vi "Day 2 (Part Two).vi"() -> ()   [LabVIEW 2021]
panel:
  out "Score":i32
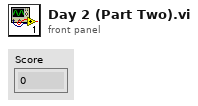
[diagram p1: front panel]
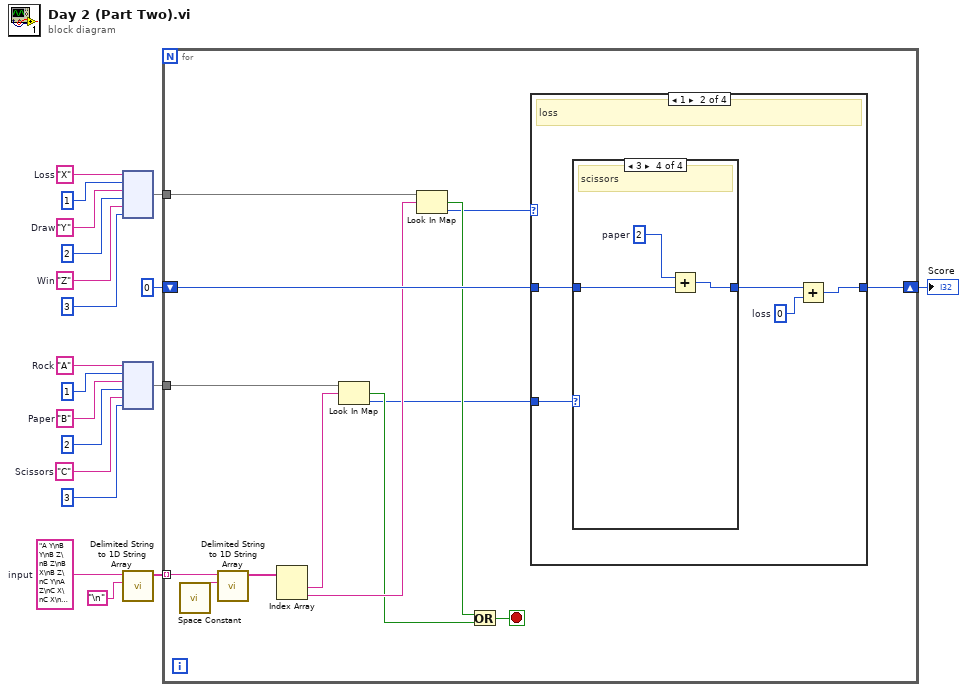
[diagram p0: block diagram]
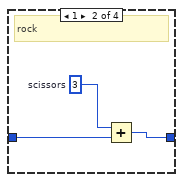
[diagram p4: hidden frame]
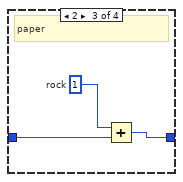
[diagram p5: hidden frame]
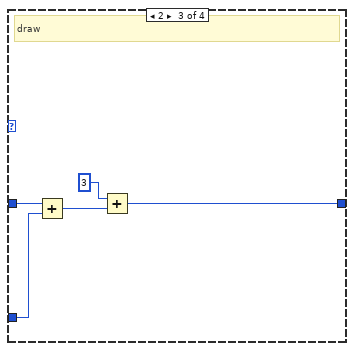
[diagram p6: hidden frame]
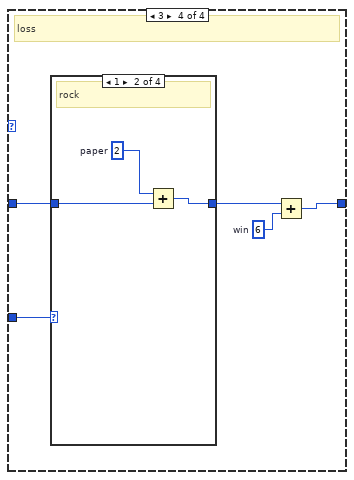
[diagram p7: hidden frame]
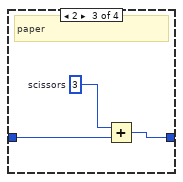
[diagram p9: hidden frame]
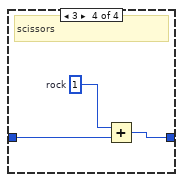
[diagram p10: hidden frame]
diagram:
  w1 = "A Y\nB Y\nB Z\nB Z\nB X\nB Z\nC Y\nA Z\nC X\nC X\nB Z\nB Z\nB Z\nA X\nB Z\nB Z\nA Y\nB Z\nA Z\nB X\nB Z\nA X\nA X\nB Z\nA Y\nA Z\nB Z\nA Y\nA Z\nB Z\nA Z\nB Z\nB Z\nC Y\nB Z\nB Z\nA X\nC X\nB Z\nA X\nB Z\nC X\nA X\nB Z\nA X\nA X\nC X\nB Z\nB Z\nB Z\nC Y\nC Y\nA X\nB Z\nC X\nB Z\nA X\nA Y\nB Z\nB Z\nB Z\nB Z\nB Z\nB X\nB Z\nB Z\nB Z\nB X\nA X\nA X\nB Z\nA Y\nC Y\nC Y\nA Y\nA X\nB Z\nA Y\nA Z\nA X\nA X\nA Y\nC Y\nB Z\nB Z\nC X\nB Z\nA Y\nA X\nB Z\nB Z\nA X\nA X\nA X\nB Z\nA Y\nB Z\nA Z\nC Y\nB Z\nB Z\nB Z\nC Y\nA Y\nC Y\nB Z\nA X\nB Z\nA X\nB Z\nC Y\nB Z\nB Z\nB Z\nC X\nB Z\nA X\nB Z\nB Z\nB Z\nA X\nA X\nB X\nC Y\nB Z\nB Z\nB Z\nA X\nB Z\nA X\nB Z\nA X\nA Z\nA X\nB Z\nA X\nC Y\nA X\nB Z\nA X\nC Y\nB Z\nB Z\nA X\nA X\nB Z\nC Y\nB Y\nB Z\nB Z\nB Z\nB X\nB Z\nB Z\nB Z\nA X\nB Z\nC Y\nC Y\nA Z\nA X\nB Z\nB Z\nB Y\nB Z\nB Z\nC Y\nB Z\nB Y\nB Z\nC Y\nB Z\nB Z\nC X\nC X\nC X\nB Z\nA Z\nA X\nC Y\nA Z\nB Z\nB Z\nB Z\nB Z\nA X\nA X\nB Z\nB Z\nA Z\nA X\nA X\nB Z\nC Y\nA X\nA Z\nA Y\nA Y\nA X\nB Z\nA X\nA Z\nB Z\nC X\nB Z\nC X\nC Y\nB Z\nB Z\nB Z\nB Z\nB Z\nC Y\nA X\nC Y\nA X\nB Y\nB Y\nA X\nA X\nB Z\nB Z\nC X\nA Z\nC Y\nA X\nA X\nA Y\nA X\nA X\nB Z\nA Z\nB Z\nB Z\nB Z\nA Z\nA X\nB Z\nB Z\nC Y\nB Z\nB Z\nB Z\nA X\nA X\nB Z\nB Z\nB Z\nB Z\nB Z\nB Z\nA X\nC X\nA X\nA X\nC Y\nA X\nB Z\nC Y\nB Z\nB Z\nB Z\nA X\nB Z\nC Y\nB Z\nA X\nA X\nB Z\nA X\nA X\nB Z\nA Z\nB X\nA X\nA X\nB Z\nC Y\nA Y\nA X\nC X\nB Z\nA X\nB Z\nB Z\nA X\nB Z\nA Z\nC Y\nB Z\nB Z\nA X\nA X\nB X\nA X\nB Z\nB Z\nC X\nA X\nC X\nA X\nB Z\nB Z\nA X\nA Z\nB Z\nB X\nA X\nA Y\nB Z\nB Z\nB Z\nC X\nC Y\nB Z\nB Z\nC Z\nB X\nC Y\nC Z\nB Z\nB Z\nA X\nB Z\nC X\nB Z\nB Z\nA Z\nA X\nC X\nB Z\nB Z\nA X\nC Y\nA X\nB X\nC Z\nB Z\nB Z\nA X\nB Z\nA Y\nB Z\nB Z\nA X\nB Z\nC Y\nC Y\nA X\nC Y\nC X\nC X\nA X\nB Z\nC Y\nB Z\nC X\nB Z\nA Z\nB Z\nA Z\nB X\nB Z\nA Z\nA X\nB Z\nB Z\nB Z\nA X\nA X\nA X\nB Z\nA X\nB Z\nB X\nA Y\nB Z\nA X\nB Z\nB Z\nB Z\nA X\nB Z\nC X\nA Y\nA X\nA Z\nC Y\nC Y\nA X\nC Y\nB Z\nA X\nB Z\nC Y\nB X\nA Z\nB Z\nB Z\nB X\nB Z\nB Z\nB Z\nA Y\nA Y\nC Y\nA Z\nA X\nB Z\nB Z\nA X\nA X\nA X\nB Z\nA X\nB Z\nB Y\nA X\nA X\nA X\nB Z\nB Z\nB Z\nC Y\nA X\nA X\nA X\nA X\nA X\nA X\nC Y\nA Z\nC X\nB Z\nB Z\nC Z\nA X\nA X\nB Z\nA X\nB X\nB Z\nB Z\nC X\nB Z\nA Z\nA X\nB Z\nA Z\nB Z\nB Y\nA X\nC Y\nA X\nB Z\nB Z\nB Z\nA Z\nC Y\nC Z\nA X\nB Z\nB Z\nB X\nA X\nB Z\nA X\nB Z\nB Z\nC Z\nB Z\nA X\nC Y\nC X\nA Z\nC X\nA X\nA X\nA X\nB Z\nB Y\nC Y\nB Z\nB Z\nC Y\nB Z\nA X\nB Z\nA Z\nA X\nB Z\nA Y\nA X\nA X\nB X\nB Z\nB Z\nB Z\nB Z\nC Z\nB Y\nA X\nA X\nB Z\nB Z\nB Z\nC Z\nB Z\nB Z\nA Y\nA Z\nB Z\nA X\nC Y\nB Z\nA Z\nC Z\nB Z\nC X\nB Z\nB Z\nA X\nB Z\nA X\nB Z\nC Y\nA X\nB Z\nA Z\nB Z\nC Y\nA X\nC X\nA X\nA X\nB Z\nB Z\nB X\nB Z\nC X\nC Y\nA Z\nB Z\nC Y\nB Z\nC Y\nB Y\nA Y\nB Z\nA X\nB Z\nA Z\nB Z\nA X\nC X\nB Z\nB X\nC Y\nA Z\nA X\nB Z\nB Z\nB Z\nA Z\nC Y\nC Y\nB Z\nA Y\nA X\nA X\nA Y\nC Y\nA Y\nB Z\nB Z\nB Z\nA Z\nB Z\nA Z\nB Z\nA X\nA Z\nB Z\nC Y\nB Z\nA X\nA X\nA X\nA Z\nA Z\nB Z\nC Y\nB Z\nA X\nB Z\nB Z\nA Z\nB Z\nB Z\nA X\nB Z\nB Z\nB X\nA X\nB Z\nB Z\nA Z\nA X\nB X\nA X\nB Z\nA X\nB Z\nA X\nB Z\nC Y\nB Z\nC Z\nC X\nB Z\nB Z\nB Z\nC Y\nC X\nB Z\nB Z\nB Z\nB Z\nA Y\nA Y\nC Y\nA X\nC X\nB X\nA X\nC X\nA Y\nB X\nA X\nA Z\nB Z\nB X\nB Y\nB Z\nB Z\nB X\nB Z\nC Y\nB Z\nA X\nA X\nA X\nB Z\nA X\nB Z\nA X\nB Z\nB Z\nB Z\nB Z\nA X\nC Y\nA X\nB Z\nB Z\nB Z\nA X\nB Z\nB Z\nC Z\nA X\nA Z\nB Z\nC Y\nB Z\nB Z\nB Z\nB Z\nA Z\nB Z\nB Z\nB Z\nC Y\nA X\nB X\nC Y\nA X\nC Z\nB Z\nC Y\nC Y\nB Z\nA X\nB Z\nC Z\nA X\nA Z\nB Z\nA Z\nB Z\nB X\nB Z\nA Z\nB Z\nC Y\nC Z\nB Z\nA X\nB Z\nA X\nA X\nB Z\nB Z\nB Z\nB Z\nA X\nA Z\nA X\nB X\nB Z\nA Y\nA Y\nB Z\nA X\nB Z\nB Z\nA Y\nC X\nB Z\nB Z\nB Z\nC X\nB Z\nC X\nA X\nB Z\nC Y\nA X\nA X\nA X\nC Z\nA X\nA X\nA Y\nB Z\nB Z\nB Z\nB Z\nB Z\nC X\nC Y\nB Z\nB Z\nC X\nB Z\nB Z\nB Z\nC Y\nC Y\nA Z\nA X\nB Z\nA X\nB X\nB Z\nB Z\nC Y\nB Z\nA X\nB X\nA Z\nA Z\nB Z\nA X\nC X\nA X\nB Z\nB Z\nB Z\nA X\nA Z\nC X\nB Z\nA X\nA Z\nA Z\nA Z\nA Z\nC Y\nB X\nB X\nC Z\nB X\nC Z\nA X\nA Y\nB Z\nB X\nA Y\nA Z\nB X\nA X\nA X\nC Z\nA Z\nB Z\nC X\nB Z\nB Z\nC X\nB Z\nC X\nA X\nA Y\nA X\nB Z\nA X\nB Z\nC Y\nB Z\nB Z\nB Z\nB Z\nB Z\nB Z\nB Z\nB Z\nB Z\nA X\nB Z\nA X\nB Z\nA Y\nB Z\nA X\nA Z\nB Z\nC Y\nA Z\nA X\nA Z\nC X\nB Z\nB Z\nB Z\nA X\nC X\nC Y\nB Z\nA Z\nA Z\nC X\nB Z\nC Y\nA Z\nA Z\nA Y\nB Z\nA Z\nB Z\nB Y\nC Y\nB Z\nB Z\nA Z\nA X\nB Z\nC Y\nB Z\nB Z\nB Z\nB Z\nB Z\nA X\nC Y\nB X\nC X\nB Z\nA Z\nB Z\nA X\nB Z\nB Z\nA X\nC Y\nA X\nA X\nA X\nC X\nA X\nA X\nB Z\nA Y\nA X\nB Z\nC X\nA X\nC Z\nA X\nB Z\nC X\nA X\nA X\nA X\nB Z\nC X\nB Z\nB Z\nA X\nA X\nA X\nA X\nB Z\nA X\nA X\nB Z\nB X\nA Y\nA X\nC X\nA X\nC X\nA X\nB Z\nB Z\nB Z\nB Z\nB Z\nA X\nA X\nB X\nC Y\nA Y\nC X\nC X\nC X\nB Z\nB Z\nB X\nB Z\nB Z\nC X\nB Z\nB Z\nA X\nB Z\nB Z\nB X\nA X\nA X\nC Y\nC X\nA X\nC Y\nA Y\nC X\nB Z\nA X\nA Z\nB Z\nB Z\nB X\nB Z\nB Z\nB Z\nC Y\nB X\nA X\nB Z\nA X\nB Z\nA X\nA Z\nA Y\nC Y\nB Z\nC Y\nA Z\nA Z\nB Z\nA X\nA X\nC Y\nC Y\nA X\nB Z\nA X\nC X\nC Z\nA X\nA Y\nA X\nA X\nA X\nB Z\nB Z\nB Z\nC Y\nB Z\nB Z\nC Z\nA X\nB Z\nB Z\nA X\nA X\nB Z\nB Z\nB Z\nA Y\nB X\nA Z\nA Z\nB Z\nA X\nB Z\nB Y\nA Y\nA X\nC Y\nA Z\nB Z\nC X\nC X\nA X\nB Z\nA X\nA X\nA Z\nB Z\nA Z\nA Z\nB Z\nB Z\nA Y\nB Z\nC Y\nC X\nB Z\nA X\nA X\nB Z\nB Z\nA X\nA X\nC Y\nB Z\nA Z\nA X\nB Z\nC Y\nB Z\nA X\nA X\nB X\nA X\nB Z\nC Y\nB Z\nA Y\nB Z\nB Z\nB Z\nB X\nA X\nB Z\nC Y\nB Z\nB Z\nB Z\nA Z\nC Y\nC Y\nC Y\nA X\nA Z\nA X\nB Z\nA X\nB Z\nA X\nC Y\nB Z\nB Z\nA X\nB Z\nA X\nA X\nB Z\nB Z\nA X\nA X\nC X\nB Z\nA Y\nA X\nA X\nB Z\nC Y\nC X\nC X\nB Y\nA Z\nB Z\nA Z\nA X\nB Z\nC Y\nB Z\nA X\nA Z\nB Z\nA X\nA Y\nA X\nB Z\nB Z\nB Y\nB Z\nA X\nB Z\nB Z\nB Z\nC Y\nA X\nB Z\nB Z\nA X\nA X\nA X\nB Z\nA Y\nB Z\nA Z\nA X\nB Z\nC X\nB Z\nA X\nA Z\nA Z\nB Z\nA X\nB Z\nB Z\nB Z\nB Z\nC Y\nA Y\nA Z\nA X\nA Y\nB Z\nB Z\nB Z\nC Y\nC Y\nB Z\nA Y\nA Z\nA X\nB Z\nA Z\nB Z\nA X\nC Y\nB Z\nB Z\nB Z\nB Z\nB Z\nC X\nA Z\nB Z\nA Z\nB Z\nA X\nB Z\nA X\nA Y\nB Z\nB X\nB Z\nA Y\nB Z\nA Z\nB Z\nB Z\nA X\nA Z\nA Z\nB X\nB Z\nA X\nB X\nA X\nA Z\nA X\nC X\nB Z\nC X\nA X\nC X\nA X\nA X\nA Z\nA Z\nB Z\nA Z\nB X\nB Z\nB Z\nA X\nB Z\nB Z\nA X\nB Z\nB Z\nB Z\nB Z\nB Z\nC X\nA X\nC Y\nB Z\nB Z\nA Y\nB X\nB Z\nA Z\nB Z\nB Z\nC Y\nB Z\nA X\nA Z\nB Z\nA Z\nB Z\nB Z\nA X\nB Z\nA Z\nA Z\nA Z\nC X\nA Z\nB Z\nC Y\nB Z\nA Z\nB Z\nA X\nA X\nA X\nA Z\nA X\nB Z\nB Z\nB Z\nB Z\nA Y\nA X\nC Y\nC Z\nB Z\nA Z\nA X\nB Z\nB X\nB Z\nA X\nB Z\nB Z\nC Y\nA X\nB Z\nB Z\nC X\nC X\nB Z\nB Y\nA Y\nA X\nC Y\nA X\nA X\nB Z\nB Z\nB Z\nB Z\nA Z\nC X\nA X\nA X\nA X\nA X\nA Y\nA Z\nA Y\nA Y\nB Z\nA X\nA Y\nA X\nA Z\nA Z\nA X\nB Z\nB Z\nC Y\nA X\nB Z\nC Y\nB Z\nB Z\nA X\nB Z\nB X\nA X\nB Z\nA Y\nA Y\nB X\nB Z\nB Z\nC X\nA X\nB Z\nA X\nB X\nB Z\nA X\nB Z\nA X\nB X\nA X\nA X\nC X\nA X\nA X\nB Z\nA X\nA X\nA Y\nB Z\nB Z\nC Y\nB Z\nA X\nB Z\nB Z\nA Z\nA X\nB Z\nA Y\nB Z\nC Y\nA Z\nA X\nA Y\nC Y\nA X\nA Y\nC X\nB Z\nA X\nA Y\nA X\nB Z\nA Z\nB Z\nB Z\nC Y\nA X\nC Y\nA Z\nB Z\nB Z\nA X\nA X\nB X\nB Z\nC Y\nB Z\nB Y\nA X\nB Z\nA X\nC X\nB Z\nA Y\nA X\nB Z\nC Y\nA Z\nB Z\nA X\nA X\nA Y\nA Z\nC X\nB Z\nB Z\nB Z\nA Z\nB Z\nC Y\nB Z\nB Z\nB Z\nB Z\nB X\nB Z\nA X\nB Z\nB Z\nA X\nC X\nC Y\nB Z\nB Z\nA X\nB Z\nA X\nA X\nA Y\nB Z\nA Z\nB Z\nC Y\nB Z\nA X\nA Y\nC Y\nB Y\nA Y\nA X\nC Y\nA X\nA Z\nA X\nB Z\nA Z\nB Z\nA X\nB Z\nC Y\nA X\nB Z\nB X\nB Z\nA X\nA X\nA X\nB Z\nA Z\nA Z\nB Z\nA X\nB Z\nB Z\nA X\nA X\nB Z\nB Z\nA X\nB Z\nB X\nB Z\nC Y\nA Z\nB X\nA X\nB Z\nB Z\nA X\nB Z\nA X\nB Z\nB X\nB X\nA X\nB Z\nB Z\nB Z\nB Z\nA Y\nB Z\nB Z\nA X\nC X\nB Z\nB Z\nB Z\nB Z\nB Z\nA X\nC X\nA Y\nA X\nA X\nB Z\nC Y\nC X\nB Z\nA X\nA Y\nB Z\nA X\nB Z\nC Y\nB Z\nA X\nB Z\nA Y\nB X\nA X\nB Z\nA X\nB Z\nA X\nB Z\nA X\nC X\nC X\nA X\nB Z\nA Y\nB Z\nB Z\nA X\nA X\nB Z\nB Z\nB Z\nA X\nA X\nA X\nC Y\nA Y\nB Z\nB Z\nB Z\nB Z\nA X\nA X\nB Z\nB Z\nC Y\nA X\nA X\nB Z\nA X\nA Y\nA X\nB Z\nB Z\nB Z\nA X\nB Z\nA X\nB Z\nA X\nA X\nB Z\nA Y\nA Z\nB Y\nA X\nA Z\nB Z\nB Z\nA Z\nA X\nA X\nB Z\nA X\nB Z\nA X\nC X\nA Z\nA X\nB Z\nB Z\nA X\nA Z\nC X\nB Z\nB Z\nA X\nB Z\nB Z\nA X\nB Z\nB Z\nB Z\nA Y\nA Z\nB Z\nB Z\nA X\nB Z\nB Z\nB X\nC X\nB Z\nB Z\nB Z\nA X\nA X\nA Z\nB Z\nC X\nB Y\nA Y\nB Z\nB Z\nA X\nA X\nA Z\nB Z\nB Z\nB Z\nA X\nA Z\nA X\nB Z\nB Z\nA Z\nB Z\nA Y\nA Z\nC Y\nB Z\nB Z\nB Z\nB Z\nA Z\nA Z\nA Y\nB Z\nA X\nA X\nB Z\nA Z\nB Z\nB Z\nB X\nC Y\nB Z\nC Y\nB Z\nA X\nC Z\nB Z\nA X\nA X\nB Z\nA Z\nA X\nB Z\nA Z\nA X\nC Z\nC X\nB Z\nB Z\nB Z\nB Z\nB Z\nC Y\nA X\nB Z\nC Y\nA X\nB Z\nB Z\nA Z\nA Z\nB Z\nC Y\nA X\nC X\nB Z\nB Z\nB Z\nB Z\nA X\nB Z\nA X\nB Z\nA Y\nB Z\nB Z\nB Z\nB Z\nB Z\nC Y\nB Z\nB Z\nA X\nA X\nA X\nA Z\nB Z\nA Y\nC Z\nA Z\nB Z\nB Z\nB Z\nA X\nB X\nC Y\nC X\nC Y\nB Z\nB Z\nB Z\nB Z\nA Y\nB Z\nA X\nC X\nA X\nB X\nC X\nB Z\nB Z\nA X\nA X\nC Y\nC Y\nA X\nB Z\nC Y\nA Y\nA Z\nA Y\nB Z\nB Z\nB Z\nA Y\nB Z\nA Z\nA X\nB Z\nC X\nA Z\nB Z\nA X\nC X\nA X\nC Y\nB X\nB Z\nB Z\nA X\nC Y\nA X\nB Z\nC X\nA Z\nA Y\nB Z\nA Z\nB Z\nB Z\nB Z\nB Z\nA X\nA X\nB Z\nA Z\nC Y\nA Y\nA X\nA X\nB Z\nC Z\nB Z\nA Z\nB X\nC X\nB Z\nB Z\nA X\nA Z\nA X\nA Z\nA X\nB Z\nB Z\nC Y\nB Z\nB Z\nB Z\nB Z\nA Z\nB Z\nB X\nB Z\nB Z\nB Z\nB Z\nC X\nC X\nA X\nB Z\nB Z\nB Z\nB Z\nB Z\nB Z\nA X\nC X\nB Z\nB Z\nA Y\nB Z\nA X\nC Y\nB Z\nC Y\nB Z\nA Y\nB Z\nB Z\nB Z\nA X\nA X\nA X\nB Z\nC Y\nB Z\nA Z\nA Y\nA Z\nA Y\nB Z\nA X\nB X\nB Z\nA X\nB Z\nA Y\nA X\nB Z\nA X\nA X\nA Y\nA Y\nA X\nA X\nA X\nB Z\nB Z\nB Z\nA X\nB Z\nA X\nB Z\nA X\nB Y\nB Y\nA X\nB Z\nC X\nA Z\nC Y\nA X\nB Z\nB Z\nB Z\nC Y\nB X\nC Y\nB Z\nB Z\nB Z\nA Z\nB Z\nB Z\nB Z\nC Y\nB Z\nB Z\nA X\nA Z\nA Y\nC Y\nB Z\nB Z\nA X\nB Z\nB Z\nA X\nA X\nB Z\nB Y\nB Z\nB Z\nA Z\nB Z\nB Z\nA X\nB Z\nA X\nC X\nC X\nA X\nC Y\nB Z\nB Z\nB Z\nA X\nC Y\nB Z\nB Z\nB Z\nB Z\nB Z\nB Z\nB Z\nB Z\nB Z\nB Z\nC Y\nC X\nB Z\nB Z\nB Z\nC Y\nA Y\nC Y\nA X\nB X\nB Z\nA X\nC X\nB Z\nA Z\nC X\nC X\nB Z\nB Z\nA Z\nB Z\nB X\nB Z\nB Z\nB Z\nA X\nC X\nB Z\nA X\nC Y\nB Z\nB Z\nC X\nB X\nA X\nB Z\nC X\nC X\nB Z\nB X\nA X\nB Z\nA Y\nB Z\nA Z\nA X\nB Z\nA X\nA X\nB Z\nB Z\nA X\nB Z\nA X\nA X\nC Y\nB Z\nA X\nC Y\nB Z\nB Z\nA X\nA Y\nC Y\nB Z\nA X\nB Z\nA X\nA X\nB Z\nB Z\nC Y\nB Z\nA X\nA X\nA X\nA X\nA Z\nB Z\nB Z\nC X\nC X\nB Z\nB Z\nC Y\nB Z\nA Y\nB Z\nA X\nC X\nA Z\nB Z\nB Z\nB Z\nC Y\nA X\nB Z\nB Z\nC Y\nB Z\nC Y\nB Z\nA Z\nB Z\nA X\nB Z\nC Y\nC Y\nA X\nA X\nA Z\nB Z\nC Y\nC Y\nA X\nB Z\nB Z\nA X\nB Z\nB Z\nB Z\nB Z\nB X\nB Y\nA X\nB Z\nB Z\nB Z\nC Y\nA X\nA Y\nB Z\nA Z\nA Z\nB X\nA X\nC Y\nB Z\nB Z\nA Z\nB Z\nC X\nC X\nA Z\nB Z\nA X\nB Z\nA X\nB Z\nB Z\nB X\nA X\nA Z\nB X\nA X\nB Z\nA X\nA X\nA Z\nA Y\nB Z\nA Y\nC Y\nC X\nB Z\nB Z\nA X\nA X\nB Z\nB Z\nB Z\nA Z\nC X\nA X\nB Z\nB Z\nA X\nB Z\nB Z\nB Z\nA X\nA Z\nB Z\nA X\nB Z\nA X\nB Z\nB Z\nA X\nC Y\nA X\nC X\nA Z\nB X\nA Y\nA Y\nB Z\nB Z\nB Z\nA X\nA X\nA X\nA Y\nB Z\nB Z\nB Z\nB Z\nB Z\nB Z\nB Z\nB Z\nC Y\nB Z\nB Z\nB Z\nC Y\nA X\nA Z\nB Z\nC Y\nB Z\nA Z\nA X\nB Z\nA Y\nB Z\nB Z\nA Z\nB Z\nA X\nA Z\nA Z\nB Z\nB Z\nB Z\nB Z\nA X\nA Z\nB Z\nB Z\nB Z\nB Z\nA Z\nB Z\nC X\nB Z\nB Y\nA X\nB Z\nB Z\nA X\nB Z\nA X\nA X\nA X\nA X\nB X\nB Z\nC X\nB Z\nB Z\nB Z\nA X\nB Z\nC X\nB Z\nA Z\nA X\nA X\nB Z\nB Z\nB Z\nB Z\nC X\nA X\nB Z\nB Z\nC Y\nB Z\nC Y\nB Z\nB Z\nA X\nB Z\nA X\nA Y\nB Z\nA Z\nB Z\nB Z\nA Y\nB Z\nB Z\nC Y\nA X\nA X\nA X\nA X\nB Z\nB Z\nA Y\nB Z\nA Z\nA X\nA X\nB Z\nA Y\nB Z\nB Z\nB X\nA Y\nA X\nA X\nC Y\nC X\nA X\nB Z\nB Z\nB Z\nA Y\nB Z\nC X\nC X\nC X\nB Z\nB Z\nB Z\nB Z\nB Z\nA X\nB Z\nA Y\nB Z\nA Y\nC X\nB X\nB Z\nB Z\nA X\nB X\nB Z\nB Z\nB Z\nB Z\nB Z\nA X\nB Z\nC X\nB X\nA X\nA X\nA X\nA X\nA X\nB Z\nC X\nC Y\nA X\nB Z\nC X\nA Z\nB Z\nB Z\nC Y\nA X\nA Z\nB Z\nB Z\nB Z\nB Z\nB Z\nB Z\nA X\nA X\nB X\nA X\nB Z\nA X\nB Z\nB Z\nA Z\nB Z\nB Z\nB Z\nB Z\nC X\nB Z\nA Z\nB Z\nB Z\nA Z\nA X\nC X\nB X\nC X\nA X\nB Z\nA Z\nB X\nB X\nA Z\nB Z\nB Z\nB X\nB Z\nB Z\nC X\nA Y\nA X\nA Z\nB Z\nA X\nB Z\nB Z\nB Z\nB Z\nA X\nA X\nC Y\nB Z\nB Z\nB Z\nA Z\nC X\nC Y\nB Y\nB Z\nB Z\nA X\nC Y\nA Z\nB Z\nB Z\nB Z\nB Z\nB Z\nC X\nB Z\nA X\nC X\nA X\nA Z\nC Y\nC X\nB Z\nB Z\nA Y\nA Z\nA Z\nA X\nA Z\nA Z\nC Y\nB Z\nB Z\nB Z\nB Z\nA Z\nA X\nA Y\nC X\nA X\nB Z\nB Z\nB Z\nA X\nB Z\nB Z\nA Z\nB Z\nA X\nB Z\nA X\nA Y\nB Z\nA X\nA Z\nB Z\nA X\nB Z\nC X\nB Z\nB Z\nC X\nA Y\nB Z\nA Z\nC X\nC Z\nC X\nB Z\nB Z\nB Z\nA X\nB Z\nC X\nA X\nA Y\nA X\nA Z\nC Y\nA X\nB Z\nB Z\nC Z\nA X\nB Z\nB Z\nA X\nA Z\nB Z\nA Y\nB Z\nC X\nA X\nA X\nB Z\nB Z\nB Z\nB X\nC X\nB Z\nB Z\nA X\nA X\nA Z\nB Z\nB Z\nA Z\nC Y\nC Z\nB Z\nA X\nA X\nA X\nC Y\nA X\nA X\nA X\nA Z\nB Z\nA Y\nB Z\nC X\nB Z\nA X\nC X\nB Z\nA Y\nA X\nB Z\nB Z\nB Z\nA X\nA Y\nB Z\nA X\nB Z\nB Z\nB Z\nB Z\nA X\nA X\nB Z\nC X\nB X\nA Z\nB Z\nB Z\nB Z\nB Z\nB Z"  # input
  w9 = "Z"  # Win
  w11 = "Y"  # Draw
  w6 = "X"  # Loss
  w14 = "C"  # Scissors
  w12 = "B"  # Paper
  w17 = "A"  # Rock
  n1 = node(w6, 1 ("value"), w11, 2 ("value"), w9, 3 ("value")) -> (w4:map{string, i32})
  n2 = node(w17, 1 ("value"), w12, 2 ("value"), w14, 3 ("value")) -> (w5:map{string, i32})
  n3 = call <vilib>:"Delimited String to 1D String Array.vi"("delimiter"="\n", "delimited string"=w1) -> ("string array"=w18:string[])  [unwired: 9 in]
  n4 = for {
    tunnel: w18 -> [w33] mode=indexing
    tunnel: w4 -> [w31]
    tunnel: w5 -> [w30]
    shift-right: [w28] -> w2
    shift-left: 0 -> [w29]
    stop <- w22 stop-if-true
    n5 = call <vilib>:"Space Constant.vi"() -> ("String"=w32:string)
    n6 = call <vilib>:"Delimited String to 1D String Array.vi"("delimiter"=w32, "delimited string"=w33) -> ("string array"=w27:string[])  [unwired: 9 in]
    n7 = Index Array(array=w27) -> (element #1=w25:string, element #2=w26:string)  [unwired: 2 in]
    n8 = Look In Map(map=w30, key=w25) -> (key not found?=w24:bool, value=w21:i32)  [unwired: 1 in]
    n9 = Look In Map(map=w31, key=w26) -> (key not found?=w23:bool, value=w20:i32)  [unwired: 1 in]
    n10 = Or(x=w23, y=w24) -> (x .or. y?=w22:bool)
    n11 = case shown="1" w20 {
      tunnel: w21 -> [_ w38 w51 w58]
      tunnel: w29 -> [w34 w39 w52 w59]
      tunnel: [w34 w36 w54 w56] -> w28
      frame Default {
      }
      frame 1 {
        w35 = 0  # loss
        # "loss"
        n12 = case shown="3" w38 {
          tunnel: w39 -> [w40 w43 w46 w49]
          tunnel: [w40 w42 w45 w48] -> w37
          frame Default {
          }
          frame 1 {
            w41 = 3  # scissors
            # "rock"
            n13 = Add(x=w41, y=w43) -> (x+y=w42:i32)
          }
          frame 2 {
            w44 = 1  # rock
            # "paper"
            n14 = Add(x=w44, y=w46) -> (x+y=w45:i32)
          }
          frame 3 {
            w47 = 2  # paper
            # "scissors"
            n15 = Add(x=w47, y=w49) -> (x+y=w48:i32)
          }
        }
        n16 = Add(x=w37, y=w35) -> (x+y=w36:i32)
      }
      frame 2 {
        # "draw"
        n17 = Add(x=w52, y=w51) -> (x+y=w50:i32)
        n18 = Add(x=3, y=w50) -> (x+y=w54:i32)
      }
      frame 3 {
        w55 = 6  # win
        # "loss"
        n19 = case shown="1" w58 {
          tunnel: w59 -> [w60 w63 w66 w69]
          tunnel: [w60 w62 w65 w68] -> w57
          frame Default {
          }
          frame 1 {
            w61 = 2  # paper
            # "rock"
            n20 = Add(x=w61, y=w63) -> (x+y=w62:i32)
          }
          frame 2 {
            w64 = 3  # scissors
            # "paper"
            n21 = Add(x=w64, y=w66) -> (x+y=w65:i32)
          }
          frame 3 {
            w67 = 1  # rock
            # "scissors"
            n22 = Add(x=w67, y=w69) -> (x+y=w68:i32)
          }
        }
        n23 = Add(x=w57, y=w55) -> (x+y=w56:i32)
      }
    }
  }
  "Score" <- w2
